vi "KeyboardControl2_RT_Main.vi"() -> ()   [LabVIEW 2014]
uses:
  <vilib>/myRIO/Instrument Drivers/Onboard IO/PWM/typedefs/PWM Reference.ctl
  <vilib>/myRIO/Common/Instrument Driver Framework/Utilities/typedefs/myRIO Generic Hardware Reference.ctl
  <vilib>/myRIO/Common/Instrument Driver Framework/Utilities/typedefs/Hardware Version Enum.ctl
  <vilib>/myRIO/Common/Instrument Driver Framework/Utilities/typedefs/myRIO v1.0 Reference.ctl
  <vilib>/myRIO/Common/Instrument Driver Framework/Utilities/typedefs/Generic FPGA Reference.ctl
  <vilib>/myRIO/Common/Instrument Driver Framework/myRIO v1.0/PWM/typedefs/PWM Channels Enum.ctl
  <vilib>/myRIO/Instrument Drivers/Onboard IO/PWM/typedefs/PWM Configuration.ctl
  <vilib>/userdefined/High Color/nirio_resource_hc.ctl
  <vilib>/myRIO/Instrument Drivers/Onboard IO/AI/typedefs/AI Reference.ctl
  <vilib>/myRIO/Common/Instrument Driver Framework/myRIO v1.0/AI/typedefs/AI Channels List.ctl
  <vilib>/myRIO/Common/Instrument Driver Framework/myRIO v1.0/AI/typedefs/AI Channels Enum.ctl
  <vilib>/myRIO/Common/Instrument Driver Framework/Utilities/typedefs/Analog Scaling Constants List.ctl
  <vilib>/myRIO/Common/Instrument Driver Framework/Utilities/typedefs/Analog Scaling Constants.ctl
  <vilib>/myRIO/Common/Instrument Driver Framework/myRIO v1.0/PWM/vis/myRIO v1.1 Open PWM.vi
  <vilib>/myRIO/Common/Instrument Driver Framework/myRIO v1.0/AI/vis/myRIO v1.1 Open AI.vi
  <vilib>/myRIO/Common/Instrument Driver Framework/Utilities/vis/Validate Channels.vi
  <vilib>/myRIO/Common/Instrument Driver Framework/myRIO v1.0/PWM/vis/myRIO v1.0 Reserve PWM.vi
  <vilib>/myRIO/Instrument Drivers/Onboard IO/PWM/vis/Set Duty Cycle and Frequency.vi
  <vilib>/myRIO/Common/Instrument Driver Framework/myRIO v1.0/AI/vis/myRIO v1.0 Reserve AI.vi
  <vilib>/myRIO/Common/Instrument Driver Framework/myRIO v1.0/DIO/vis/myRIO v1.1 Open DIO.vi
  <vilib>/myRIO/Common/Instrument Driver Framework/myRIO v1.0/PWM/vis/myRIO v1.0 Close PWM.vi
  <vilib>/myRIO/Common/Instrument Driver Framework/myRIO v1.0/AI/vis/myRIO v1.0 Close AI.vi
  <vilib>/myRIO/Common/Instrument Driver Framework/myRIO v1.0/DIO/vis/myRIO v1.0 Close DIO.vi
  <vilib>/myRIO/Common/Instrument Driver Framework/myRIO v1.0/PWM/vis/myRIO v1.0 Build MUX Configuration PWM.vi
  <vilib>/myRIO/Common/Instrument Driver Framework/myRIO v1.0/Resource Manager/vis/myRIO v1.0 Reserve Channel List.vi
  <vilib>/myRIO/Common/Instrument Driver Framework/myRIO v1.0/AI/vis/myRIO v1.0 Build MUX Configuration AI.vi
  <vilib>/myRIO/Common/Instrument Driver Framework/myRIO v1.0/DIO/vis/myRIO v1.0 Reserve DIO.vi
  <vilib>/myRIO/Common/Instrument Driver Framework/myRIO v1.0/PWM/vis/myRIO v1.0 Unreserve PWM.vi
  <vilib>/myRIO/Common/Instrument Driver Framework/myRIO v1.0/AI/vis/myRIO v1.0 Unreserve AI.vi
  <vilib>/myRIO/Common/Instrument Driver Framework/myRIO v1.0/DIO/vis/myRIO v1.0 Unreserve DIO.vi
  <vilib>/myRIO/Common/Instrument Driver Framework/myRIO v1.0/Resource Manager/vis/myRIO v1.0 Create Configuration List.vi
  <vilib>/myRIO/Common/Instrument Driver Framework/myRIO v1.0/Resource Manager/vis/myRIO v1.0 Reserve Channel.vi
  <vilib>/myRIO/Common/Instrument Driver Framework/myRIO v1.0/Resource Manager/vis/myRIO v1.0 Unreserve Channel.vi
  <vilib>/myRIO/Common/Instrument Driver Framework/myRIO v1.0/DIO/vis/myRIO v1.0 Build MUX Configuration DIO.vi
  <vilib>/myRIO/Common/Instrument Driver Framework/myRIO v1.0/Resource Manager/vis/myRIO v1.0 Unreserve Channel List.vi
  <vilib>/myRIO/Common/Instrument Driver Framework/myRIO v1.0/Resource Manager/vis/myRIO v1.0 Build Mutex Name.vi
  <vilib>/Utility/VariantDataType/GetNumericInfo.vi
  <vilib>/Utility/error.llb/Error Cluster From Error Code.vi
  <vilib>/myRIO/Common/Instrument Driver Framework/myRIO v1.0/myRIO v1.1 Open.vi
  <vilib>/myRIO/Common/Instrument Driver Framework/Utilities/vis/IO Manager.vi
  <vilib>/myRIO/Common/Instrument Driver Framework/Utilities/vis/Configuration Manager.vi
  <vilib>/myRIO/Common/Instrument Driver Framework/myRIO v1.0/Resource Manager/vis/myRIO v1.0 Configure IO.vi
  <vilib>/myRIO/Common/Instrument Driver Framework/myRIO v1.0/myRIO v1.0 Close.vi
  <vilib>/myRIO/Common/Instrument Driver Framework/myRIO v1.0/AI/vis/myRIO v1.0 Get Scaling Constants AI.vi
  <vilib>/myRIO/Common/Instrument Driver Framework/myRIO v1.0/PWM/vis/myRIO v1.0 Write PWM.vi
  <vilib>/myRIO/Common/Instrument Driver Framework/myRIO v1.0/PWM/vis/myRIO v1.0 Shutdown PWM.vi
  <vilib>/myRIO/Common/Instrument Driver Framework/myRIO v1.0/AI/vis/myRIO v1.0 Read AI.vi
  <vilib>/myRIO/Common/Instrument Driver Framework/myRIO v1.0/DIO/vis/myRIO v1.0 Write DIO.vi
  <vilib>/myRIO/Common/Instrument Driver Framework/myRIO v1.0/DIO/vis/myRIO v1.0 Shutdown DIO.vi
  <vilib>/myRIO/Instrument Drivers/Onboard IO/AI/vis/myRIO AI Open.xnode
  <vilib>/myRIO/Instrument Drivers/Onboard IO/PWM/vis/myRIO PWM Open.xnode
  <vilib>/myRIO/Instrument Drivers/Onboard IO/DIO/DIO.lvlib
  <vilib>/myRIO/Instrument Drivers/Onboard IO/AI/AI.lvlib
  <vilib>/myRIO/Instrument Drivers/Onboard IO/PWM/PWM.lvlib
  <vilib>/gmath/NI_Gmath.lvlib
panel:
  out "Pot Control On":bool
  out "PropmotorInput":dbl
  out "ServoInput":dbl
  in  "Pot. Degrees":dbl[](array[numeric])
  out "Volts":dbl(knob) scale=0.0..10.0
  in  "Propmotor PWM Channel":tag="C/PWM1"
  in  "Servo PWM Channel":tag="C/PWM0"
  out "Propmotor keybd":dbl
  out "ServoKeybd":dbl
  out "error out":errorcluster={"status"=FALSE, "code"=-363018, "source"=""}
  out "RT FP LED":bool
  in  "Stop":bool
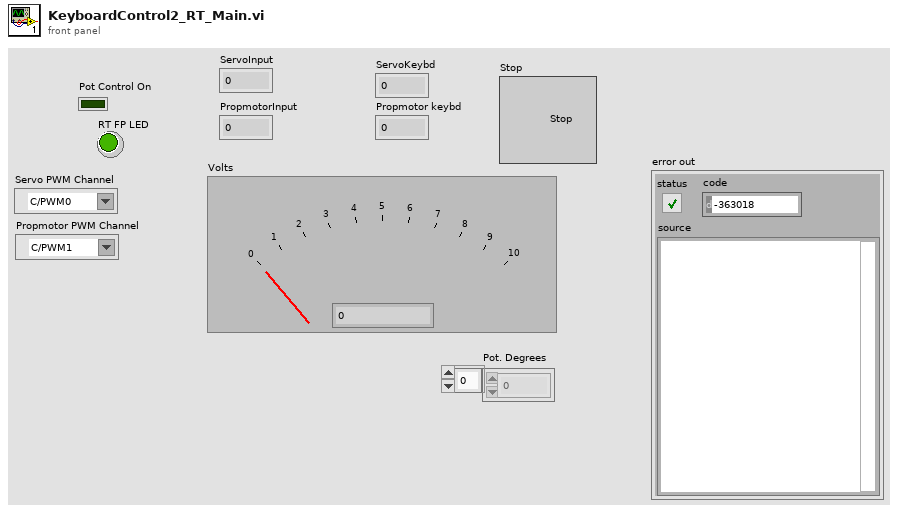
[diagram p1: front panel]
types:
  T1 = typedef "nirio_resource_hc.ctl" = tag
  T2 = typedef "Hardware Version Enum.ctl" = enum16{"Unknown", "myRIO-1900", "myRIO-1950"}
  T3 = typedef "PWM.lvlib/PWM Reference.ctl" = cluster{"myRIO Reference":T4, "PWM Channels Enum":T7, "PWM Configuration":T8}
  T4 = typedef "myRIO Generic Hardware Reference.ctl" = cluster{"myRIO Model":T2, "myRIO Hardware Reference":T5}
  T5 = typedef "myRIO v1.0 Reference.ctl" = cluster{"Generic FPGA Reference":T6, "Allow multiple opens":bool}
  T6 = typedef "Generic FPGA Reference.ctl" = refnum<k20>
  T7 = typedef "PWM Channels Enum.ctl" = enum16{"Not Connected", "C/PWM0", "C/PWM1", "A/PWM0", "A/PWM1", "A/PWM2", "B/PWM0", "B/PWM1", "B/PWM2"}
  T8 = typedef "PWM.lvlib/PWM Configuration.ctl" = cluster{"Frequency":dbl, "Duty Cycle":dbl}
  T9 = typedef "AI.lvlib/AI Reference.ctl" = cluster{"myRIO Reference":T4, "AI Channels List":T10, "AI Scaling Constants List":T12}
  T10 = typedef "AI Channels List.ctl" = T11[]
  T11 = typedef "AI Channels Enum.ctl" = enum16{"Not Connected", "AudioIn/Left", "AudioIn/Right", "C/AI0", "C/AI1", "A/AI0", "A/AI1", "A/AI2", "A/AI3", "B/AI0", "B/AI1", "B/AI2", "B/AI3"}
  T12 = typedef "Analog Scaling Constants List.ctl" = T13[]
  T13 = typedef "Analog Scaling Constants.ctl" = cluster{"LSB Weight (Volts)":dbl, "Offset (Volts)":dbl, "Signed?":bool}
  T14 = typedef "DIO.lvlib/DIO Reference.ctl" = cluster{"myRIO Reference":T4, "DIO Channels List":T15}
  T15 = typedef "DIO Channels List.ctl" = T16[]
  T16 = typedef "DIO Channels Enum.ctl" = enum16{"Not Connected", "C/DIO0", "C/DIO1", "C/DIO2", "C/DIO3", "C/DIO4", "C/DIO5", "C/DIO6", "C/DIO7", "A/DIO0", "A/DIO1", "A/DIO2", "A/DIO3", "A/DIO4", "A/DIO5", "A/DIO6", "A/DIO7", "A/DIO8", "A/DIO9", "A/DIO10", "A/DIO11", "A/DIO12", "A/DIO13", "A/DIO14", "A/DIO15", "B/DIO0", "B/DIO1", "B/DIO2", "B/DIO3", "B/DIO4", "B/DIO5", "B/DIO6", "B/DIO7", "B/DIO8", "B/DIO9", "B/DIO10", "B/DIO11", "B/DIO12", "B/DIO13", "B/DIO14", "B/DIO15", "LED0", "LED1", "LED2", "LED3", "Button0"}
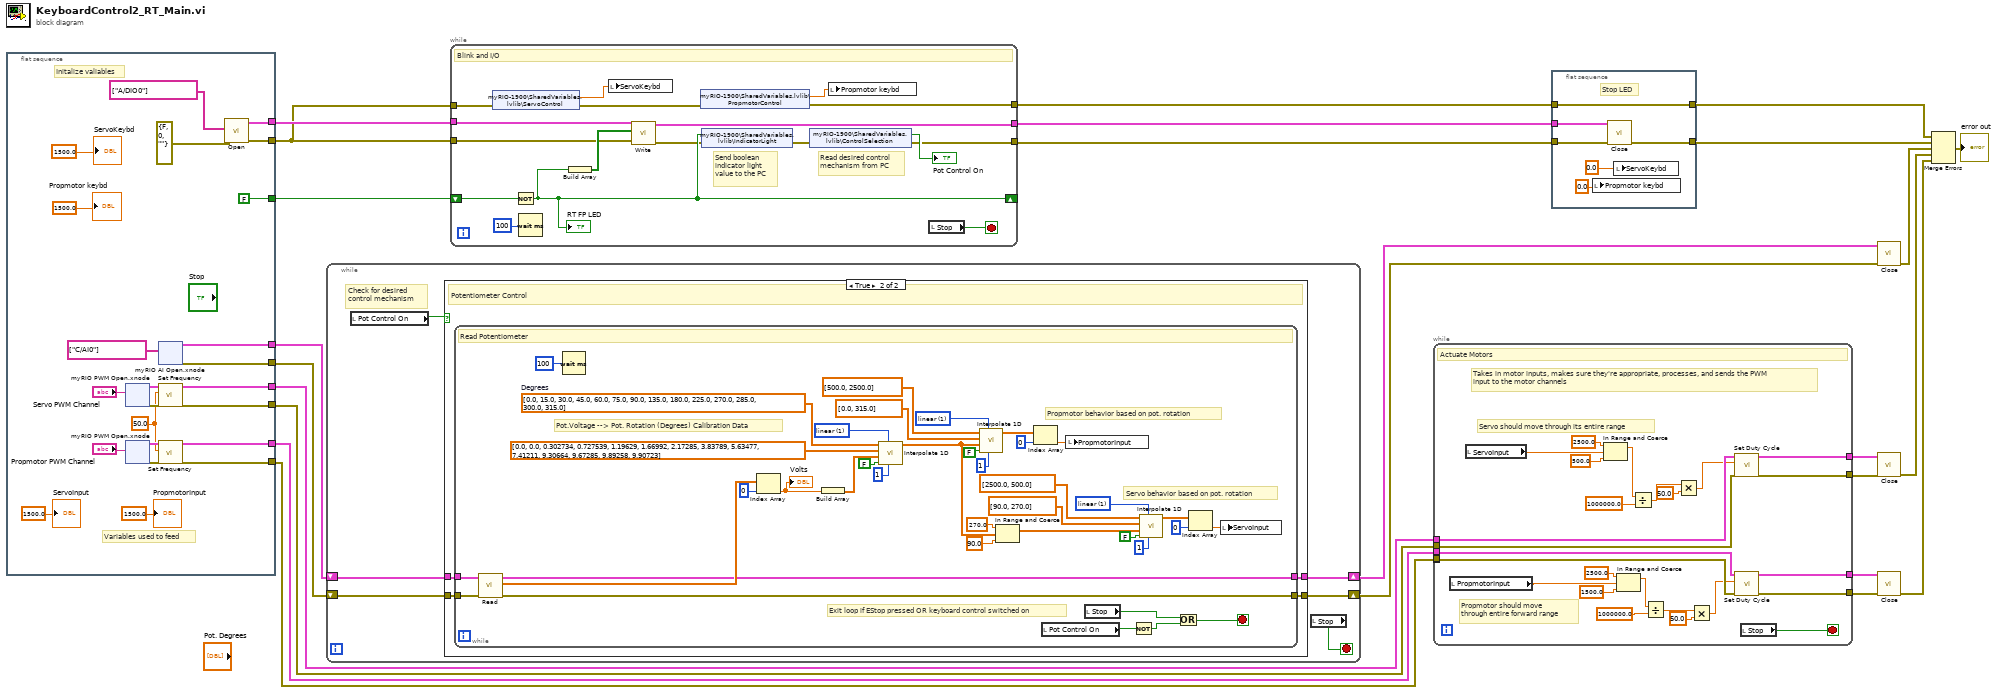
[diagram p0: block diagram]
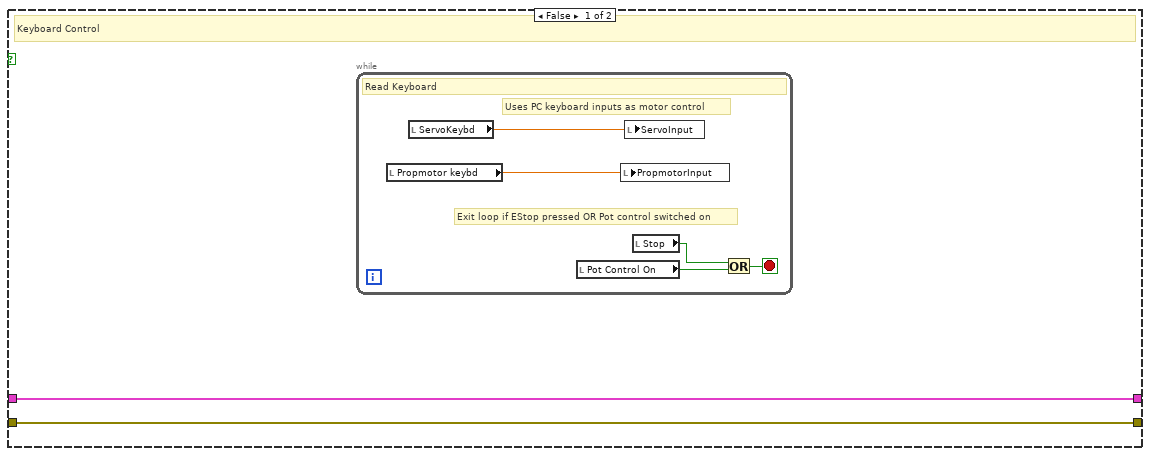
[diagram p2: hidden frame]
diagram:
  n1 = flat-sequence {
    tunnel: [FALSE] -> w24
    tunnel: [w46] -> w20
    tunnel: [w45] -> w23
    tunnel: [w32] -> w17
    tunnel: [w31] -> w16
    tunnel: [w30] -> w14
    tunnel: [w29] -> w13
    tunnel: [w28] -> w12
    tunnel: [w27] -> w15
    frame #0 {
      w33 = 50.0 ("Frequency [Hz]")
      # "Variables used to feed"
      # "Initalize valiables"
      n2 = xnode "myRIO PWM Open.xnode"("Channel Name"="Servo PWM Channel") -> ("error out"=w38:errorcluster, "PWM Ref Out"=w39:T3)  [unwired: 2 in]
      n3 = xnode "myRIO PWM Open.xnode"("Channel Name"="Propmotor PWM Channel") -> ("error out"=w35:errorcluster, "PWM Ref Out"=w36:T3)  [unwired: 2 in]
      n4 = xnode "myRIO AI Open.xnode"("Channel Names"=tag[] ["C/AI0"]) -> ("error out"=w31:errorcluster, "AI Ref Out"=w32:T9)  [unwired: 2 in]
      n5 = call <vilib>:"Set Frequency.vi"("error in (no error)"=w38, "Frequency [Hz]"=w33, "PWM Ref In"=w39) -> ("error out"=w30:errorcluster, "PWM Ref Out"=w27:T3)  [unwired: 6 in]
      n6 = call <vilib>:"Set Frequency.vi"("error in (no error)"=w35, "Frequency [Hz]"=w33, "PWM Ref In"=w36) -> ("error out"=w28:errorcluster, "PWM Ref Out"=w29:T3)  [unwired: 6 in]
      n7 = call <vilib>:"Open.vi"("error in (no error)"=errorcluster {"status"=FALSE, "code"=0, "source"=""}, "Channel Names"=tag[] ["A/DIO0"]) -> ("error out"=w46:errorcluster, "DIO Ref Out"=w45:T14)  [unwired: 8 in]
      "ServoKeybd" <- 1500.0
      "Propmotor keybd" <- 1500.0
      "ServoInput" <- 1500.0 ("ServoInput")
      "PropmotorInput" <- 1500.0 ("PropmotorInput")
    }
  }
  n8 = while {
    shift-right: [w101] -> w7
    shift-left: w17 -> [w103]
    shift-right: [w100] -> w6
    shift-left: w16 -> [w102]
    stop <- w98 stop-if-true
    # "Check for desired\ncontrol mechanism"
    n9 = local read "Pot Control On"() -> (w99:bool)
    n10 = case shown="True" w99 {
      tunnel: w103 -> [w105 w114]
      tunnel: w102 -> [w104 w113]
      tunnel: [w105 w112] -> w101
      tunnel: [w104 w111] -> w100
      frame False {
        # "Keyboard Control"
        n11 = while {
          stop <- w108 stop-if-true
          # "Exit loop if EStop pressed OR Pot control switched on"
          # "Uses PC keyboard inputs as motor control"
          # "Read Keyboard"
          n12 = local read "Propmotor keybd"() -> (w109:dbl)
          n13 = local read "ServoKeybd"() -> (w110:dbl)
          n14 = local read "Pot Control On"() -> (w106:bool)
          n15 = local write "PropmotorInput"(w109) -> ()
          n16 = local write "ServoInput"(w110) -> ()
          n17 = local read "Stop"() -> (w107:bool)
          n18 = Or(x=w107, y=w106) -> (x .or. y?=w108:bool)
        }
      }
      frame True {
        # "Potentiometer Control"
        n19 = while {
          tunnel: w114 -> [w151]
          tunnel: w113 -> [w150]
          tunnel: [w147] -> w111
          tunnel: [w146] -> w112
          stop <- w115 stop-if-true
          w124 = 1 items=["nearest", "linear", "spline", "cubic Hermite", "Lagrange"] ("method")
          w136 = 1 items=["nearest", "linear", "spline", "cubic Hermite", "Lagrange"] ("method")
          w139 = dbl[] [0.0, 15.0, 30.0, 45.0, 60.0, 75.0, 90.0, 135.0, 180.0, 225.0, 270.0, 285.0, 300.0, 315.0]  # Degrees
          w141 = 1 items=["nearest", "linear", "spline", "cubic Hermite", "Lagrange"] ("method")
          # "Exit loop if EStop pressed OR keyboard control switched on"
          # "Propmotor behavior based on pot. rotation"
          # "Servo behavior based on pot. rotation"
          # "Pot.Voltage --> Pot. Rotation (Degrees) Calibration Data"
          # "Read Potentiometer"
          n20 = call <vilib>:"Read.vi"("error in (no error)"=w150, "AI Ref In"=w151) -> ("error out"=w147:errorcluster, "Values"=w149:dbl[], "AI Ref Out"=w146:T9)  [unwired: 7 in]
          n21 = Wait (ms)(milliseconds to wait=u32 100) -> ()  [unwired: 1 out]
          n22 = Index Array(array=w149, index=0) -> (element=w144:dbl)
          "Volts" <- w144
          n23 = Build Array(w144) -> (w143:dbl[])
          n24 = call <vilib>:"Interpolate 1D.vi"("ntimes"=1, "method"=w141, "X is monotonic"=FALSE, "xi"=w143, "X"=dbl[] [0.0, 0.0, 0.302734, 0.727539, 1.19629, 1.66992, 2.17285, 3.83789, 5.63477, 7.41211, 9.30664, 9.67285, 9.89258, 9.90723] ("VoltageIn"), "Y"=w139) -> ("yi"=w122:dbl[])  [unwired: 3 in, 2 out]
          n25 = call <vilib>:"Interpolate 1D.vi"("ntimes"=1, "method"=w124, "X is monotonic"=FALSE, "xi"=w122, "X"=dbl[] [0.0, 315.0] ("X servo (degrees)"), "Y"=dbl[] [500.0, 2500.0] ("Y servo (PWM)")) -> ("yi"=w123:dbl[])  [unwired: 3 in, 2 out]
          n26 = In Range and Coerce(upper limit=270.0, x=w122, lower limit=90.0) -> (coerced(x)=w132:dbl[])  [unwired: 1 out]
          n27 = Index Array(array=w123, index=0) -> (element=w119:dbl)
          n28 = local read "Pot Control On"() -> (w118:bool)
          n29 = local write "PropmotorInput"(w119) -> ()
          n30 = local read "Stop"() -> (w117:bool)
          n31 = Not(x=w118) -> (.not. x?=w116:bool)
          n32 = call <vilib>:"Interpolate 1D.vi"("ntimes"=1, "method"=w136, "X is monotonic"=FALSE, "xi"=w132, "X"=dbl[] [90.0, 270.0] ("X servo (degrees)"), "Y"=dbl[] [2500.0, 500.0] ("Y servo (PWM)")) -> ("yi"=w131:dbl[])  [unwired: 3 in, 2 out]
          n33 = Or(x=w117, y=w116) -> (x .or. y?=w115:bool)
          n34 = Index Array(array=w131, index=0) -> (element=w120:dbl)
          n35 = local write "ServoInput"(w120) -> ()
        }
      }
    }
    n36 = local read "Stop"() -> (w98:bool)
  }
  n37 = while {
    shift-right: [w164] -> _
    shift-left: w24 -> [w169]
    tunnel: w23 -> [w165]
    tunnel: w20 -> [w155]
    tunnel: [w153] -> w22
    tunnel: [w167] -> w21
    tunnel: [w162] -> w18
    tunnel: w20 -> [w161]
    stop <- w158 stop-if-true
    # "Read desired control\nmechanism from PC"
    # "Send boolean\nindicator light\nvalue to the PC"
    # "Blink and I/O"
    n38 = shared-variable "myRIO-1900\\SharedVariables.lvlib\\ServoControl"(error in=w161) -> (w159:dbl, error out=w163:errorcluster)
    n39 = Not(x=w169) -> (.not. x?=w164:bool)
    "RT FP LED" <- w164
    n40 = Wait (ms)(milliseconds to wait=u32 100) -> ()  [unwired: 1 out]
    n41 = Build Array(w164) -> (w166:bool[])
    n42 = local write "ServoKeybd"(w159) -> ()
    n43 = call <vilib>:"Write.vi"("error in (no error)"=w155, "Values"=w166, "DIO Ref In"=w165) -> ("error out"=w156:errorcluster, "DIO Ref Out"=w167:T14)  [unwired: 6 in]
    n44 = shared-variable "myRIO-1900\\SharedVariables.lvlib\\PropmotorControl"(error in=w163) -> (w160:dbl, error out=w162:errorcluster)
    n45 = shared-variable "myRIO-1900\\SharedVariables.lvlib\\IndicatorLight"(w164, error in=w156) -> (error out=w154:errorcluster)
    n46 = shared-variable "myRIO-1900\\SharedVariables.lvlib\\ControlSelection"(error in=w154) -> (→"Pot Control On":bool, error out=w153:errorcluster)
    n47 = local write "Propmotor keybd"(w160) -> ()
    n48 = local read "Stop"() -> (w158:bool)
  }
  n49 = while {
    tunnel: w15 -> [w193]
    tunnel: w14 -> [w192]
    tunnel: w13 -> [w191]
    tunnel: w12 -> [w190]
    tunnel: [w190] -> _
    tunnel: [w189] -> w11
    tunnel: [w188] -> w10
    tunnel: [w187] -> w8
    tunnel: [w186] -> w9
    stop <- w194 stop-if-true
    # "Propmotor should move\nthrough entire forward range"
    # "Servo should move through its entire range"
    # "Takes in motor inputs, makes sure they're appropriate, processes, and sends the PWM\ninput to the motor channels"
    # "Actuate Motors"
    n50 = local read "PropmotorInput"() -> (w171:dbl)
    n51 = local read "ServoInput"() -> (w170:dbl)
    n52 = In Range and Coerce(upper limit=2500.0, x=w170, lower limit=500.0) -> (coerced(x)=w184:dbl)  [unwired: 1 out]
    n53 = In Range and Coerce(upper limit=2500.0, x=w171, lower limit=1500.0) -> (coerced(x)=w177:dbl)  [unwired: 1 out]
    n54 = Divide(x=w184, y=1000000.0) -> (x/y=w182:dbl)
    n55 = Divide(x=w177, y=1000000.0) -> (x/y=w174:dbl)
    n56 = Multiply(x=w182, y=50.0) -> (x*y=w172:dbl)
    n57 = Multiply(x=w174, y=50.0) -> (x*y=w173:dbl)
    n58 = call <vilib>:"Set Duty Cycle.vi"("error in (no error)"=w192, "Duty Cycle"=w172, "PWM Ref In"=w193) -> ("error out"=w188:errorcluster, "PWM Ref Out"=w189:T3)  [unwired: 6 in]
    n59 = call <vilib>:"Set Duty Cycle.vi"("error in (no error)"=w190, "Duty Cycle"=w173, "PWM Ref In"=w191) -> ("error out"=w187:errorcluster, "PWM Ref Out"=w186:T3)  [unwired: 6 in]
    n60 = local read "Stop"() -> (w194:bool)
  }
  n61 = flat-sequence {
    tunnel: w22 -> [w200]
    tunnel: w21 -> [w199]
    tunnel: [w198] -> w1
    tunnel: w18 -> [w197]
    tunnel: [w197] -> w2
    frame #0 {
      # "Stop LED"
      n62 = local write "Propmotor keybd"(0.0) -> ()
      n63 = call <vilib>:"Close.vi"("error in (no error)"=w200, "DIO Ref In"=w199) -> ("error out"=w198:errorcluster)  [unwired: 9 in]
      n64 = local write "ServoKeybd"(0.0) -> ()
    }
  }
  n65 = call <vilib>:"Close.vi"("error in (no error)"=w6, "AI Ref In"=w7) -> ("error out"=w5:errorcluster)  [unwired: 9 in]
  n66 = call <vilib>:"Close.vi"("error in (no error)"=w10, "PWM Ref In"=w11) -> ("error out"=w3:errorcluster)  [unwired: 9 in]
  n67 = call <vilib>:"Close.vi"("error in (no error)"=w8, "PWM Ref In"=w9) -> ("error out"=w4:errorcluster)  [unwired: 9 in]
  n68 = Merge Errors(w2, w1, w5, w3, w4) -> (→"error out":errorcluster)
